vi "Actor Core.vi"(8 "error in":errorcluster, 11 "Measurment Actor in":refnum<class "Measurment Actor.lvclass">) -> (0 "error out":errorcluster, 3 "Actor out":refnum<class "Actor.lvclass">)   [LabVIEW 2019, in "Measurment Actor.lvlib" / "Measurment Actor.lvclass"]
doc: "(<B>Filename</B>: Actor Framework.lvlib:Actor.lvclass:Actor Core.vi)\n\nReceives messages to the actor, reacts to them, and initiates any error handling that may shut the actor down.\n\nDescendant classes may override this VI to append parallel tasks for the actor to complete while it handles messages. Overrides use the Call Parent Method node."
uses:
  Measurment Actor.lvclass
  C:/Program Files (x86)/National Instruments/LabVIEW 2019/vi.lib/ActorFramework/Actor/Actor.lvclass
  <vilib>/ActorFramework/Actor/Actor.lvclass
  <vilib>/ActorFramework/Actor/Actor.lvclass/Actor.ctl
  Measurment Actor.lvclass/Measurment Actor.ctl
  GUI Actor Messages/Graph data Msg/Graph data Msg.lvclass/Graph data Msg.ctl
  <vilib>/ActorFramework/Message Enqueuer/Message Enqueuer.lvclass/Message Enqueuer.ctl
  <vilib>/ActorFramework/Message Enqueuer/Enqueue.vi
  GUI Actor Messages/Graph data Msg/Graph data Msg.lvclass
  C:/Program Files (x86)/National Instruments/LabVIEW 2019/vi.lib/ActorFramework/Message/Message.lvclass
  <vilib>/ActorFramework/Message Priority Queue/Priority Enqueue.vi
  <vilib>/measure/NI_MABase.lvlib
panel:
  out "StartStop Hl":bool
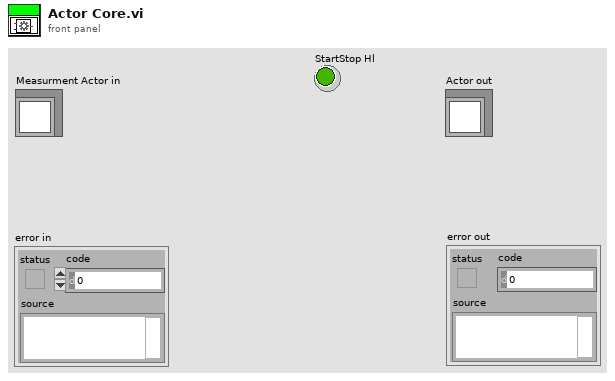
[diagram p1: front panel]
types:
  T1 = cluster{"Start Stop Hl":refnum<user-event>, "Exit":refnum<user-event>, "Amplitud":refnum<user-event>, "Frecuencia":refnum<user-event>, "Tipo de señal":refnum<user-event>}
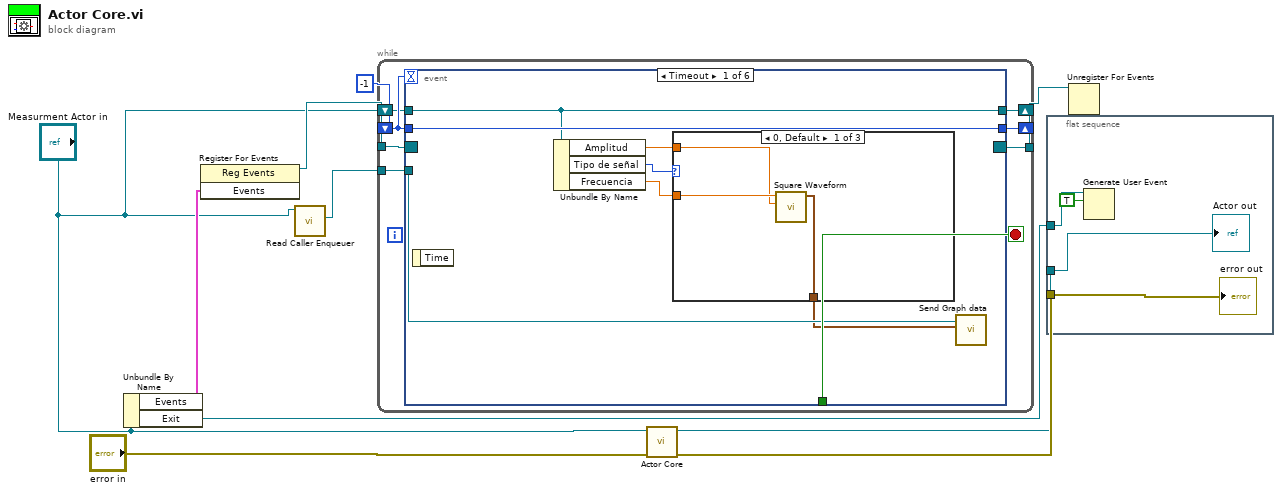
[diagram p0: block diagram]
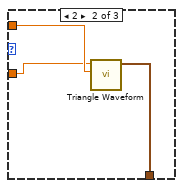
[diagram p2: hidden frame]
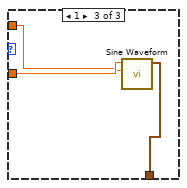
[diagram p3: hidden frame]
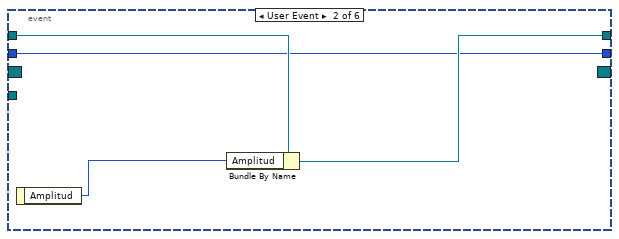
[diagram p4: hidden frame]
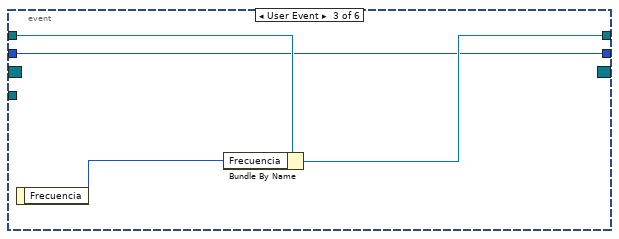
[diagram p5: hidden frame]
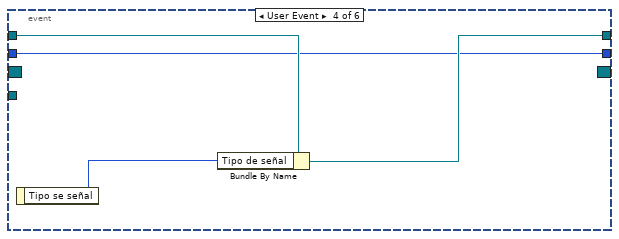
[diagram p6: hidden frame]
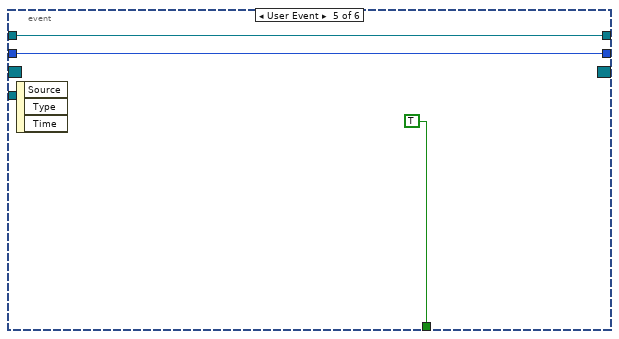
[diagram p7: hidden frame]
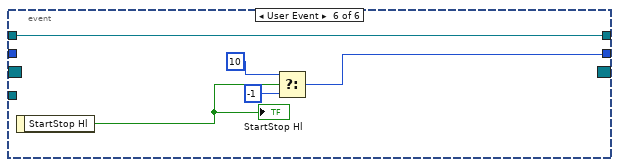
[diagram p8: hidden frame]
diagram:
  n1 = Unbundle By Name("Measurment Actor in") -> ("Events"=w6:T1, "Exit"=w3:refnum<user-event>)
  n2 = register-events(w6) -> (reference out=w5:refnum<event-registration>)  [unwired: 2 in, 1 out]
  n3 = call <vilib>:"Read Caller Enqueuer.vi"("Actor"="Measurment Actor in") -> ("Caller Enqueuer"=w2:refnum<class "Message Enqueuer.lvclass">)  [unwired: 10 in]
  n4 = while {
    shift-right: [w17] -> _
    shift-left: -1 -> [w18]
    tunnel: w5 -> [w16]
    tunnel: [w15] -> w4
    tunnel: w2 -> [w13]
    shift-right: [w11] -> _
    shift-left: "Measurment Actor in" -> [w12]
    stop <- w14 stop-if-true
    n5 = event shown="[0] Timeout" {
      selector: w16 -> [_ _ _ _ _ _]
      dyn-events: [_ _ _ _ _ _] -> w15
      timeout: w18 -> [_ _ _ _ _ _]
      tunnel: w18 -> [w25 w35 w39 w43 w48 _]
      tunnel: [w25 w35 w39 w43 w48 w51] -> w17
      tunnel: [_ _ _ _ TRUE _] -> w14
      tunnel: w13 -> [w24 _ _ _ _ _]
      tunnel: w12 -> [w23 w37 w41 w45 w47 w50]
      tunnel: [w23 w36 w40 w44 w47 w50] -> w11
      event Timeout {
        n6 = event-data() -> ()  [unwired: 1 in, 1 out]
        n7 = Unbundle By Name(w23) -> ("Amplitud"=w20:dbl, "Tipo de señal"=w22:u16, "Frecuencia"=w21:dbl)
        n8 = case shown="0, Default" w22 {
          tunnel: w21 -> [w28 w30 w34]
          tunnel: w20 -> [w27 w31 w33]
          tunnel: [w26 w29 w32] -> w19
          frame 0, Default {
            n9 = call <vilib>:"Square Waveform.vi"("amplitude"=w27, "frequency"=w28) -> ("signal out"=w26:waveform(dbl))  [unwired: 8 in, 1 out]
          }
          frame 2 {
            n10 = call <vilib>:"Triangle Waveform.vi"("amplitude"=w31, "frequency"=w30) -> ("signal out"=w29:waveform(dbl))  [unwired: 8 in, 1 out]
          }
          frame 1 {
            n11 = call <vilib>:"Sine Waveform.vi"("amplitude"=w33, "frequency"=w34) -> ("signal out"=w32:waveform(dbl))  [unwired: 8 in, 1 out]
          }
        }
        n12 = call "Send Graph data.vi"("signal out"=w19, "Message Enqueuer"=w24) -> ()  [unwired: 8 in, 2 out]
      }
      event User Event {
        n13 = event-data() -> ("Amplitud"=w38:i32)  [unwired: 1 in]
        n14 = Bundle By Name(cluster=w37, "Amplitud"=w38) -> (w36:refnum<class "Measurment Actor.lvclass">)
      }
      event User Event {
        n15 = event-data() -> ("Frecuencia"=w42:i32)  [unwired: 1 in]
        n16 = Bundle By Name(cluster=w41, "Frecuencia"=w42) -> (w40:refnum<class "Measurment Actor.lvclass">)
      }
      event User Event {
        n17 = event-data() -> ("Tipo se señal"=w46:u16)  [unwired: 1 in]
        n18 = Bundle By Name(cluster=w45, "Tipo de señal"=w46) -> (w44:refnum<class "Measurment Actor.lvclass">)
      }
      event User Event {
        n19 = event-data() -> ()  [unwired: 1 in, 3 out]
      }
      event User Event {
        n20 = event-data() -> ("StartStop Hl"=w54:bool)  [unwired: 1 in]
        "StartStop Hl" <- w54
        n21 = Select(t=10, s=w54, f=-1) -> (s? t:f=w51:i32)
      }
    }
  }
  n22 = call-parent "Actor Core.vi"("error in"="error in", "Actor in"="Measurment Actor in") -> ("error out"=w10:errorcluster, "Actor out"=w9:refnum<class "Actor.lvclass">)  [unwired: 8 in]
  n23 = flat-sequence {
    tunnel: w10 -> [w58]
    tunnel: w9 -> [w57]
    tunnel: w3 -> [w56]
    frame #0 {
      n24 = Generate User Event(user event=w56, event data cluster=TRUE ("event data")) -> ()  [unwired: 2 in, 2 out]
      "error out" <- w58
      "Actor out" <- w57
    }
  }
  n25 = Unregister For Events(event registration refnum=w4) -> ()  [unwired: 1 in, 1 out]
